vi "availableGeometry.vi"(8 "Error In":errorcluster, 11 "QScreen In":refnum<class "QScreen.lvclass">) -> (0 "Error Out":errorcluster, 2 "Value":T1, 3 "QScreen Out":refnum<class "QScreen.lvclass">)   [LabVIEW 2014, in "QScreen.lvclass"]
doc: "LabVIEW-specific documentation is not yet available. See <b>https://doc.qt.io/qt-5/qscreen.html#availableGeometry</b>"
uses:
  QScreen.lvclass
  LQ Core/QRect.ctl
  LQ Core/LQIdentity/LQIdentity.lvclass/LQIdentity.ctl
  LQ Core/LQ Core.lvlib
  LQ Core/LQIdentity/LQIdentity.lvclass
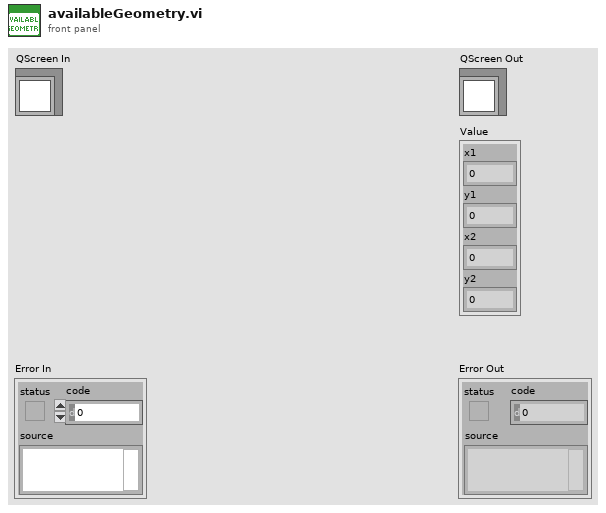
[diagram p1: front panel]
types:
  T1 = typedef "QRect.ctl" = cluster{"x1":i32, "y1":i32, "x2":i32, "y2":i32}
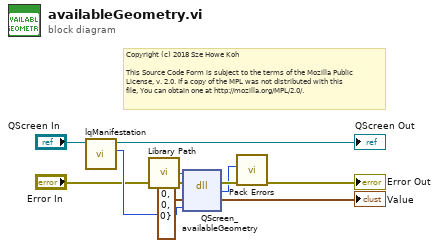
[diagram p0: block diagram]
diagram:
  # "Copyright (c) 2018 Sze Howe Koh\n\nThis Source Code Form is subject to the terms of the Mozilla Public\nLicense, v. 2.0. If a copy of the MPL was not distributed with this\nfile, You can obtain one at http://mozilla.org/MPL/2.0/."
  n1 = call "lqManifestation.vi"("LQIdentity in"="QScreen In") -> ("Manifestation"=w5:u64, "LQIdentity out"=→"QScreen Out":refnum<class "QScreen.lvclass">)  [unwired: 9 in]
  n2 = call "Library Path.vi"() -> ("Library Path"=w6:path)
  n3 = dll-call lib="?" fn="QScreen_availableGeometry"(path in=w6, error in="Error In", "_retVal"=T1 {"x1"=0, "y1"=0, "x2"=0, "y2"=0} ("retVal"), "_instance"=w5) -> (error out=w3:errorcluster, w1:i32, "_retVal"=→"Value":T1)  [unwired: 2 in, 1 out]
  n4 = call "Pack Errors.vi"("Error In"=w3, "Error Code"=w1) -> ("Error Out"=→"Error Out":errorcluster)  [unwired: 9 in]
